vi "Date-Time String.vi"() -> (0 "Date Time":string)   [LabVIEW 2009]
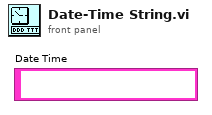
[diagram p1: front panel]
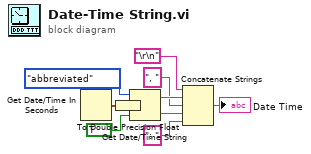
[diagram p0: block diagram]
diagram:
  n1 = Get Date/Time In Seconds() -> (seconds since 1Jan1904=w1:timestamp)
  n2 = To Double Precision Float(number=w1) -> (double precision float=w10:dbl)
  n3 = Get Date/Time String(date format (0)=enum16{"short", "long", "abbreviated"}."abbreviated", seconds (now)=w10, want seconds? (F)=TRUE) -> (date string=w8:string, time string=w7:string)
  n4 = Concatenate Strings("\r\n", w8, ", " ("Substring"), w7, ": ") -> (→"Date Time":string)
